vi "Periodic Tasks.vi"(8 "error in":errorcluster) -> ()   [LabVIEW 2014]
doc: "This VI runs in parallel to other tasks. It can contain as many user-defined periodic loops as you need. These can carry out PID or other sorts of timed response."
uses:
  <vilib>/Rock Robotics/WPI/Joystick/WPI_JoystickGetSetRefNum.vi
  <vilib>/Rock Robotics/WPI/RobotDrive/WPI_RobotDriveGetSetRefNum.vi
  <vilib>/Rock Robotics/WPI/Ultrasonic/WPI_SonarMB1010AnalogRefNum Registry Get.vi
  <vilib>/Rock Robotics/WPI/Ultrasonic/WPI_SonarMB1010AnalogGetRange.vi
  <vilib>/Rock Robotics/Network Tables/SD Write Number.vi
  <vilib>/Rock Robotics/Network Tables/SD Write Numeric Array.vi
  Robot Global Data.vi
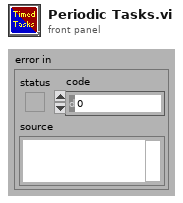
[diagram p1: front panel]
types:
  T1 = typedef "WPI_JoystickDevRef.ctl" = cluster{"Device":T2}
  T2 = typedef "WPI_JoystickDeviceEnum.ctl" = enum16{"USB 0", "USB 1", "USB 2", "USB 3", "USB 4", "USB 5"}
  T3 = typedef "WPI_RobotDriveDevRef.ctl" = cluster{"DevStatus":errorcluster, "Motors[]":T4[], "Square Inputs":bool, "Max Output":dbl}
  T4 = typedef "WPI_MotorControlDeviceRef.ctl" = cluster{"DeviceStatus":errorcluster, "Type":T5, "PWM":cluster{"Controller":T6, "PWM Channel":T7, "DeadBand":T8}, "CAN":cluster{"Device Number":u8, "Control Mode":T9, "Semaphore":T10, "Max Vout":dbl, "TalonSRX Control Mode":T11}, "Invert":bool, "TransformRef":T12, "InvTransformRef":T12}
  T5 = typedef "WPI_MotorControlType.ctl" = enum16{"PWM", "CAN", "CANTalonSRX"}
  T6 = typedef "FPGA_TypedefDigitalModule.ctl" = enum16{"Controller 1"}
  T7 = typedef "FPGA_DIOPWMChannel.ctl" = enum8{"PWM 0", "PWM 1", "PWM 2", "PWM 3", "PWM 4", "PWM 5", "PWM 6", "PWM 7", "PWM 8", "PWM 9", "PWM MXP 0", "PWM MXP 1", "PWM MXP 2", "PWM MXP 3", "PWM MXP 4", "PWM MXP 5", "PWM MXP 6", "PWM MXP 7", "PWM MXP 8", "PWM MXP 9", "Invalid"}
  T8 = typedef "WPI_PWMDeadband.ctl" = cluster{"Name":string, "maxPositivePwm":i32, "minPositivePwm":i32, "centerPwm":i32, "maxNegativePwm":i32, "minNegativePwm":i32, "angularRange":u16}
  T9 = typedef "WPI_CANJaguar_ControlMode.ctl" = enum8{"Percent VBus", "Current", "Speed", "Position", "Voltage"}
  T10 = typedef "Semaphore RefNum" = refnum<k1>
  T11 = typedef "WPI_CANTalonSRX_APIControlMode.ctl" = enum8{"Percent VBus", "Speed", "Position", "Slave", "Unchanged / Invalid"}
  T12 = typedef "WPI_PWMTransform_ConPane.ctl" = refnum<vi>
  T13 = cluster{"JoystickDevRef":T1, "RobotDriveDevRef":T3}
  T14 = typedef "WPI_AccelerometerDevRef.ctl" = cluster{"DevStatus":errorcluster, "Controller":T15, "Scaling":T16, "Analog Channels":T17, "I2C Bus":T19, "SPI Bus":T20, "Accel Range":T21, "ADXL345 Axes":T22, "Handle":i32, "Device Address":u8, "Accel Type":enum16{"Analog", "ADXL345 I2C", "ADXL345 SPI", "Internal"}}
  T15 = typedef "FPGA_TypedefAnalogModule.ctl" = enum16{"Controller 1"}
  T16 = typedef "WPI_AccelerometerScaling.ctl" = cluster{"Gain (VoltsPerG)":dbl, "Center Voltage":dbl}
  T17 = typedef "WPI_AccelerometerAnalogChannels.ctl" = cluster{"X-Axis":T18, "Y-Axis":T18, "Z-Axis":T18}
  T18 = typedef "FPGA_AIChannel.ctl" = enum8{"AI 0", "AI 1", "AI 2", "AI 3", "AI MXP 0", "AI MXP 1", "AI MXP 2", "AI MXP 3", "Invalid"}
  T19 = typedef "i2c_bus.ctl" = enum16{"I2C On-Board", "I2C MXP", "Invalid"}
  T20 = typedef "spi_bus.ctl" = enum16{"SPI On-Board, CS0", "SPI On-Board, CS1", "SPI On-Board, CS2", "SPI On-Board, CS3", "SPI MXP", "Invalid"}
  T21 = typedef "ADXL345 Range.ctl" = u8
  T22 = typedef "WPI_AccelerometerADXL345 Axes.ctl" = cluster{"X-Axis":bool, "Y-Axis":bool, "Z-Axis":bool}
  T23 = typedef "WPI_PotentiometerDevRef.ctl" = cluster{"DevStatus":errorcluster, "Controller":T15, "Analog Channel":T18, "Invert Output":bool}
  T24 = typedef "WPI_SonarMB1010AnalogDeviceRef.ctl" = cluster{"AIDeviceRef":T25, "Scaling factor (V/in)":dbl, "Average Bits":u8}
  T25 = typedef "WPI_AnalogChannelDevRef.ctl" = cluster{"DevStatus":errorcluster, "Controller":T15, "Analog Channel":T18}
  T26 = cluster{"X-Axis":dbl, "Y-Axis":dbl, "Z-Axis":dbl}
  T27 = cluster{"Accelerations":cluster{"X-Axis":dbl, "Y-Axis":dbl, "Z-Axis":dbl}, "Normalized Value":dbl, "Distance":dbl, "Distance":dbl}
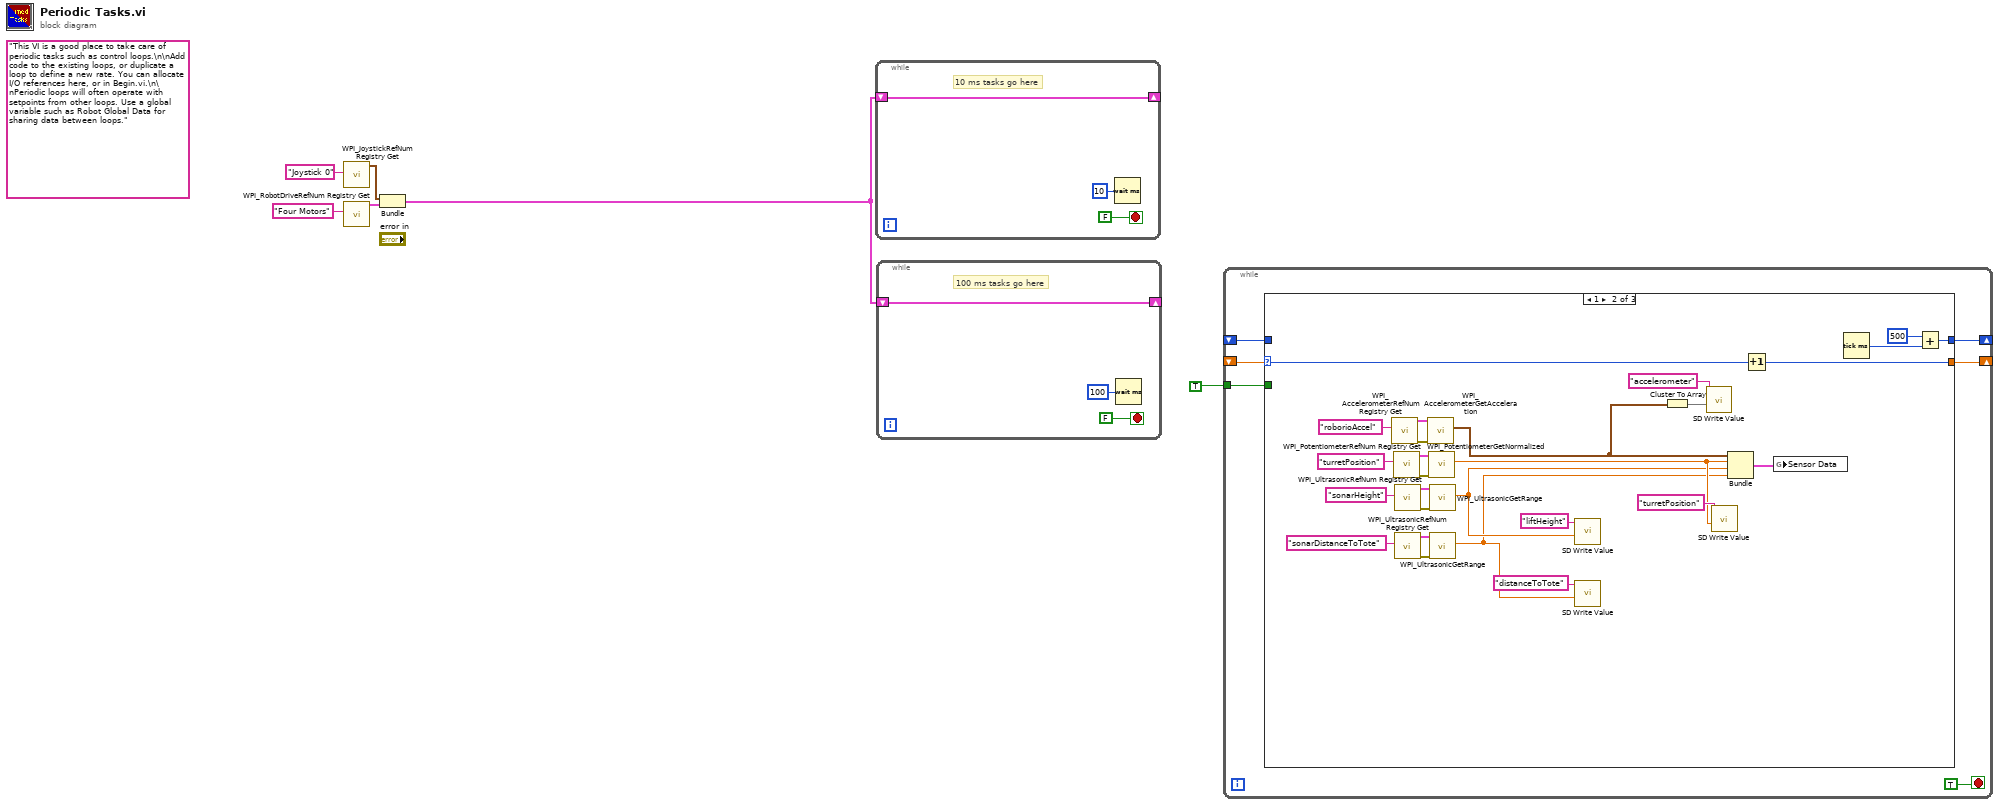
[diagram p0: block diagram]
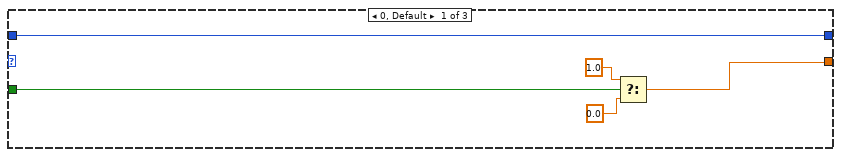
[diagram p2: hidden frame]
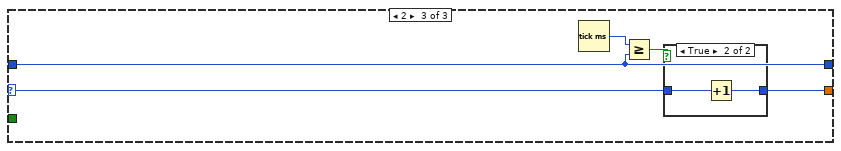
[diagram p3: hidden frame]
diagram:
  (unwired) "This VI is a good place to take care of periodic tasks such as control loops.\n\nAdd code to the existing loops, or duplicate a loop to define a new rate. You can allocate I/O references here, or in Begin.vi.\n\nPeriodic loops will often operate with setpoints from other loops. Use a global variable such as Robot Global Data for sharing data between loops."
  n1 = call <vilib>:"WPI_JoystickRefNum Registry Get.vi"("refnum name"="Joystick 0") -> ("JoystickDevRef"=w4:T1)  [unwired: 1 in, 9 out]
  n2 = call <vilib>:"WPI_RobotDriveRefNum Registry Get.vi"("refnum name"="Four Motors") -> ("RobotDriveDevRef"=w3:T3)  [unwired: 1 in, 9 out]
  n3 = Bundle("JoystickDevRef"=w4, "RobotDriveDevRef"=w3) -> (w2:T13)  [unwired: 1 out]
  n4 = while {
    shift-right: [w7] -> _
    shift-left: w2 -> [w7]
    stop <- FALSE stop-if-true
    # "10 ms tasks go here"
    n5 = Wait (ms)(milliseconds to wait=u32 10) -> ()  [unwired: 1 out]
  }
  n6 = while {
    shift-right: [w10] -> _
    shift-left: w2 -> [w10]
    stop <- FALSE stop-if-true
    # "100 ms tasks go here"
    n7 = Wait (ms)(milliseconds to wait=u32 100) -> ()  [unwired: 1 out]
  }
  n8 = while {
    shift-right: [w17] -> _
    shift-left: _ -> [w16]
    shift-right: [w15] -> _
    shift-left: _ -> [w14]
    tunnel: TRUE ("Switch Pressed") -> [w13]
    stop <- TRUE stop-if-true
    n9 = case shown="1" w16 {
      selector: w16 -> [_ w50 w54]
      tunnel: [w21 w49 w53] -> w17
      tunnel: [w20 w48 w51] -> w15
      tunnel: w14 -> [w20 _ w51]
      tunnel: w13 -> [w19 _ _]
      frame 0, Default {
        n10 = Select(t=1.0, s=w19, f=0.0) -> (s? t:f=w21:dbl)
      }
      frame 1 {
        n11 = call <vilib>:"WPI_AccelerometerRefNum Registry Get.vi"("refnum name"="roborioAccel") -> ("error out"=w32:errorcluster, "AccelerometerDevRef"=w33:T14)  [unwired: 9 in]
        n12 = call <vilib>:"WPI_PotentiometerRefNum Registry Get.vi"("refnum name"="turretPosition") -> ("error out"=w35:errorcluster, "PotDevRef"=w36:T23)  [unwired: 9 in]
        n13 = call-poly <vilib>:"WPI_UltrasonicRefNum Registry Get.vi"("refnum name"="sonarHeight") -> ("error out"=w29:errorcluster, "SonarMB1010AnalogDevRef"=w30:T24)  [unwired: 9 in]
        n14 = call-poly <vilib>:"WPI_UltrasonicRefNum Registry Get.vi"("refnum name"="sonarDistanceToTote") -> ("error out"=w26:errorcluster, "SonarMB1010AnalogDevRef"=w27:T24)  [unwired: 9 in]
        n15 = call <vilib>:"WPI_AccelerometerGetAcceleration.vi"("error in"=w32, "AccelerometerDevRef"=w33) -> ("Accelerations"=w44:T26)  [unwired: 7 in, 2 out]
        n16 = call <vilib>:"WPI_PotentiometerGetNormalized.vi"("error in"=w35, "PotDevRef"=w36) -> ("Normalized Value"=w41:dbl)  [unwired: 7 in, 2 out]
        n17 = call-poly <vilib>:"WPI_UltrasonicGetRange.vi"("error in"=w29, "SonarMB1010AnalogDevRef"=w30) -> ("Distance"=w39:dbl)  [unwired: 7 in, 2 out]
        n18 = call-poly <vilib>:"WPI_UltrasonicGetRange.vi"("error in"=w26, "SonarMB1010AnalogDevRef"=w27) -> ("Distance"=w24:dbl)  [unwired: 7 in, 2 out]
        n19 = call-poly <vilib>:"SD Write Value.vi"("Numeric"=w39, "Name"="liftHeight") -> ()  [unwired: 8 in, 2 out]
        n20 = call-poly <vilib>:"SD Write Value.vi"("Numeric"=w24, "Name"="distanceToTote") -> ()  [unwired: 8 in, 2 out]
        n21 = Cluster To Array(cluster=w44) -> (array=w45:dbl[])
        n22 = call-poly <vilib>:"SD Write Value.vi"("Numeric Array"=w45, "Name"="accelerometer") -> ()  [unwired: 8 in, 2 out]
        n23 = call-poly <vilib>:"SD Write Value.vi"("Numeric"=w41, "Name"="turretPosition") -> ()  [unwired: 8 in, 2 out]
        n24 = Bundle("Accelerations"=w44, "Normalized Value"=w41, "Distance"=w39, "Distance"=w24) -> (w38:T27)  [unwired: 1 in]
        n25 = Increment(x=w50) -> (x+1=w49:i32)
        n26 = global write "Robot Global Data.vi" "Sensor Data"(w38) -> ()
        n27 = Tick Count (ms)() -> (millisecond timer value=w47:u32)
        n28 = Add(x=u32 500, y=w47) -> (x+y=w48:u32)
      }
      frame 2 {
        n29 = Tick Count (ms)() -> (millisecond timer value=w52:u32)
        n30 = Greater Or Equal?(x=w52, y=w51) -> (x >= y?=w55:bool)
        n31 = case shown="True" w55 {
          tunnel: [w56 w57] -> w53
          tunnel: w54 -> [w56 w58]
          frame False {
          }
          frame True {
            n32 = Increment(x=w58) -> (x+1=w57:i32)
          }
        }
      }
    }
  }
